vi "Auto Size Cluster.vi"(6 "Variant in":variant, 7 "Shift Pressed?":bool, 8 "error in (no error)":errorcluster, 10 "QD Combo Box Ref":refnum<vi>, 11 "QD Launch VI Ref":refnum<vi>) -> (0 "error out":errorcluster, 4 "Variant out":variant)   [LabVIEW 2019]
doc: "Connects compatible terminals between multiple selected diagram objects. This shortcut will wire compatible data types between the objects in a left-to-right fashion. If [Shift] is also pressed, LabVIEW will perform a diagram cleanup of the selected objects after wiring them together.\n\nDefault Shortcut - [W]"
panel:
  in  "Enum":enum16{""}(ring)
  in  "Undo Name":string="Wire Multiple Objects Together"
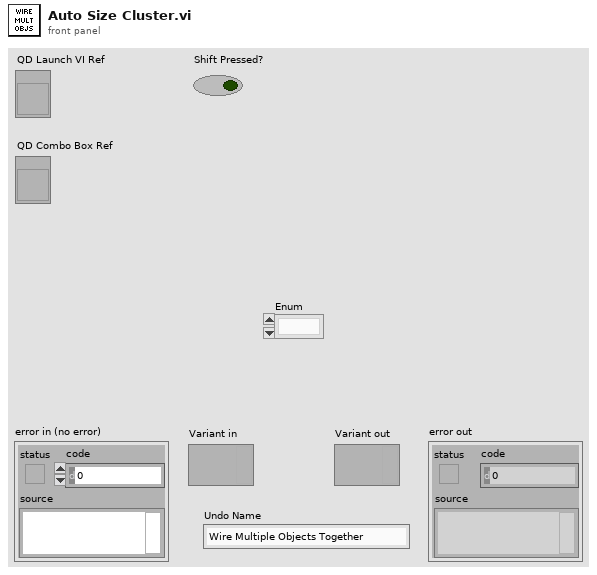
[diagram p1: front panel]
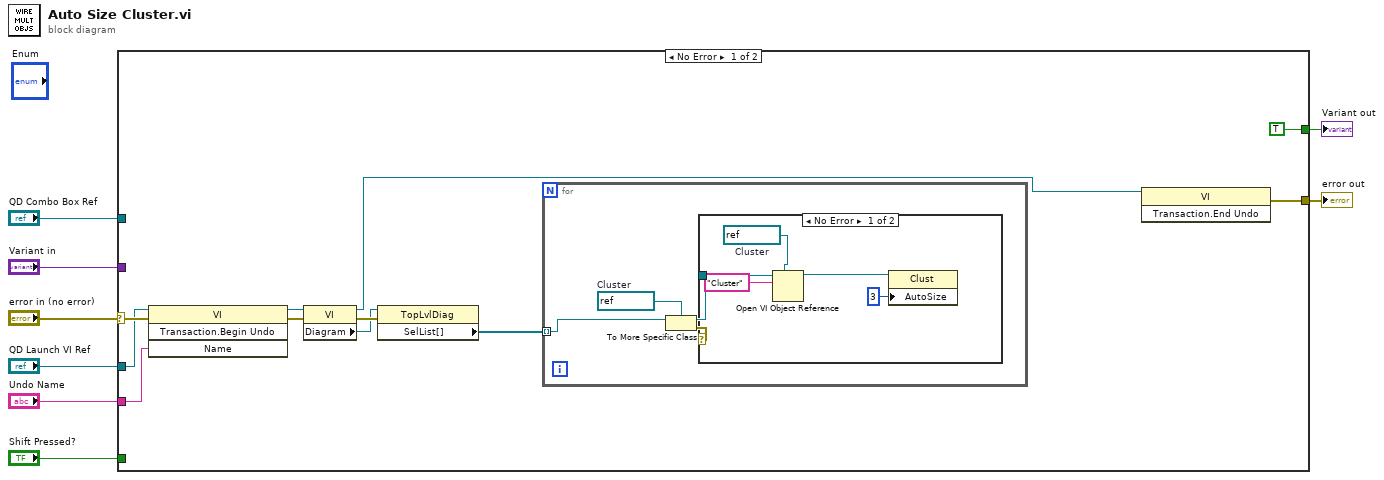
[diagram p0: block diagram]
diagram:
  n1 = case shown="No Error" "error in (no error)" {
    selector: "error in (no error)" -> [w19 w29]
    tunnel: [w14 w29] -> w7
    tunnel: "QD Launch VI Ref" -> [w18 _]
    tunnel: "Shift Pressed?" -> [_ _]
    tunnel: "QD Combo Box Ref" -> [_ _]
    tunnel: "Variant in" -> [_ _]
    tunnel: "Undo Name" -> [w17 _]
    tunnel: [TRUE _] -> w1
    frame No Error {
      n2 = invoke class="VI" method="Transaction.Begin Undo"(reference=w18, error in=w19, "Name"=w17) -> (reference out=w11:refnum<vi>, error out=w15:errorcluster)  [unwired: 1 in, 2 out]
      n3 = property class="VI"(reference=w11, error in=w15) -> (reference out=w9:refnum<vi>, error out=w13:errorcluster, "Diagram"=w12:refnum<vi>)
      n4 = property class="TopLvlDiag"(reference=w12, error in=w13) -> ("SelList[]"=w10:refnum<vi>[])  [unwired: 2 out]
      n5 = for {
        tunnel: w10 -> [w23] mode=indexing
        w22 = refnum<vi> refnum  # Cluster
        n6 = To More Specific Class(target class=w22, reference=w23) -> (specific class reference=w20:refnum<vi>, error out=w21:errorcluster)  [unwired: 1 in]
        n7 = case shown="No Error" w21 {
          tunnel: w20 -> [w28 _]
          frame No Error {
            w24 = refnum<vi> refnum  # Cluster
            n8 = Open VI Object Reference(7:w24, 10:"Cluster" ("name/order"), 11:w28) -> (3:w27:refnum<vi>)  [unwired: 1 in, 1 out]
            n9 = property class="Clust"(reference=w27, "AutoSize"=u32 3 ("Auto Sizing")) -> ()  [unwired: 1 in, 2 out]
          }
          frame Error {
          }
        }
      }
      n10 = invoke class="VI" method="Transaction.End Undo"(reference=w9) -> (error out=w14:errorcluster)  [unwired: 2 in, 2 out]
    }
    frame Error {
    }
  }
  "error out" <- w7
  "Variant out" <- w1
